vi "temp_selection.vi"(9 "temp_string":string[](array[string]), 10 "String":string, 11 "configuration file path":path) -> (3 "output array":string[](array[string]))   [LabVIEW 2021]
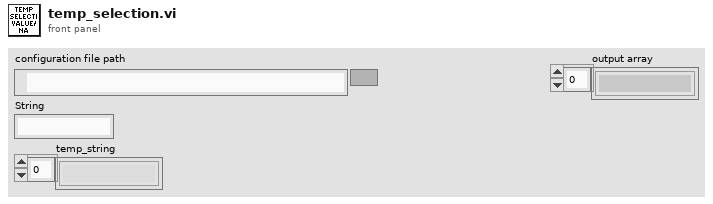
[diagram p1: front panel]
types:
  T1 = cluster{"Temp-1":bool, "Temp-2":bool, "Temp-3":bool}
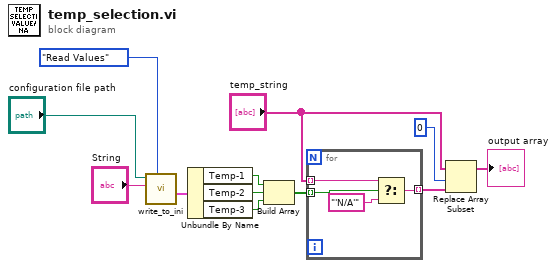
[diagram p0: block diagram]
diagram:
  n1 = call "write_to_ini.vi"("Enum"=enum16{"Write", "Read variants", "Read Values"}."Read Values", "String"="String", "configuration file path"="configuration file path") -> ("Output values"=w11:T1)  [unwired: 5 in, 3 out]
  n2 = Unbundle By Name(w11) -> ("Temp-1"=w10:bool, "Temp-2"=w9:bool, "Temp-3"=w8:bool)
  n3 = Build Array(w10, w9, w8) -> (w5:bool[])
  n4 = for {
    tunnel: w5 -> [w15] mode=indexing
    tunnel: "temp_string" -> [w16] mode=indexing
    tunnel: [w13] -> w3 mode=indexing
    n5 = Select(t=w16, s=w15, f="'N/A'") -> (s? t:f=w13:string)
  }
  n6 = Replace Array Subset(array="temp_string", new element=w3, index=0) -> (→"output array":string[])
